vi "MONTHS USING CASE STRUCTURE.vi"() -> ()   [LabVIEW 2019]
panel:
  in  "MONTH":u8
  # "MONTHS USING CASE STRUCTURE"
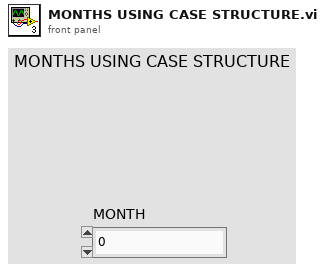
[diagram p1: front panel]
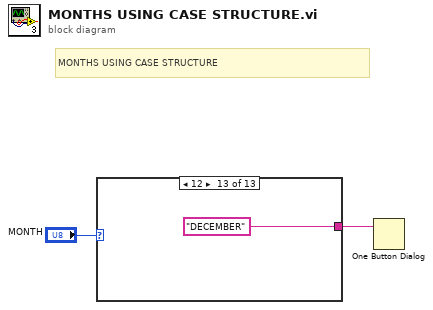
[diagram p0: block diagram]
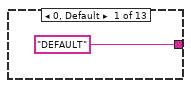
[diagram p2: hidden frame]
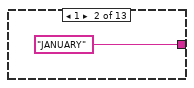
[diagram p3: hidden frame]
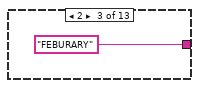
[diagram p4: hidden frame]
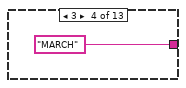
[diagram p5: hidden frame]
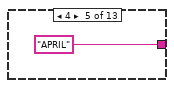
[diagram p6: hidden frame]
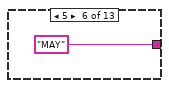
[diagram p7: hidden frame]
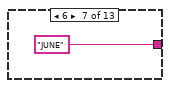
[diagram p8: hidden frame]
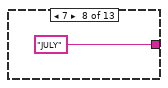
[diagram p9: hidden frame]
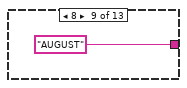
[diagram p10: hidden frame]
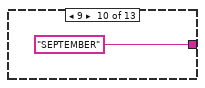
[diagram p11: hidden frame]
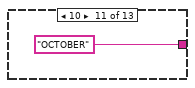
[diagram p12: hidden frame]
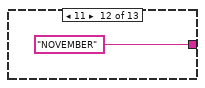
[diagram p13: hidden frame]
diagram:
  # "MONTHS USING CASE STRUCTURE"
  n1 = case shown="12" "MONTH" {
    tunnel: ["DEFAULT" ("message") "JANUARY" ("message") "FEBURARY" ("message") "MARCH" ("message") "APRIL" ("message") "MAY" ("message") "JUNE" ("message") "JULY" ("message") "AUGUST" ("message") "SEPTEMBER" ("message") "OCTOBER" ("message") "NOVEMBER" ("message") "DECEMBER" ("message")] -> w1
    frame 0, Default {
    }
    frame 1 {
    }
    frame 2 {
    }
    frame 3 {
    }
    frame 4 {
    }
    frame 5 {
    }
    frame 6 {
    }
    frame 7 {
    }
    frame 8 {
    }
    frame 9 {
    }
    frame 10 {
    }
    frame 11 {
    }
    frame 12 {
    }
  }
  n2 = One Button Dialog(message=w1) -> ()  [unwired: 1 in, 1 out]
